vi "Read Data.vi"(11 "FlukeDMM in":refnum<class "FlukeDMM.lvclass">) -> (2 "Data":string, 3 "FlukeDMM out":refnum<class "FlukeDMM.lvclass">)   [LabVIEW 2013, in "FlukeDMM.lvlib" / "FlukeDMM.lvclass"]
uses:
  <userlib>/Common/Devices/FlukeDMM/FlukeDMM/FlukeDMM.lvclass
  <userlib>/Common/Devices/FlukeDMM/FlukeDMM/FlukeDMM.lvclass/FlukeDMM.ctl
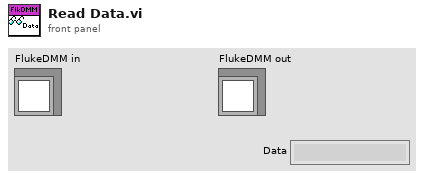
[diagram p1: front panel]
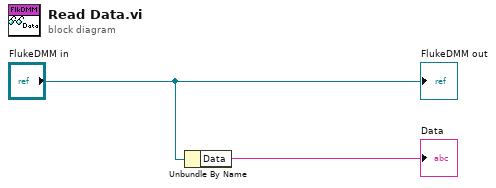
[diagram p0: block diagram]
diagram:
  n1 = Unbundle By Name("FlukeDMM in") -> ("Data"=→"Data":string)
  "FlukeDMM out" <- "FlukeDMM in"
